vi "Case Structure.vi"() -> ()   [LabVIEW 2020]
panel:
  out "Boolean":bool
  in  "Checkbox":bool
  # "Case Structure"
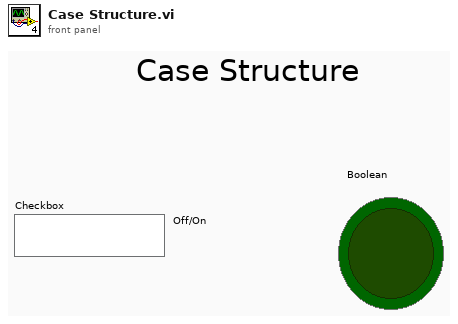
[diagram p1: front panel]
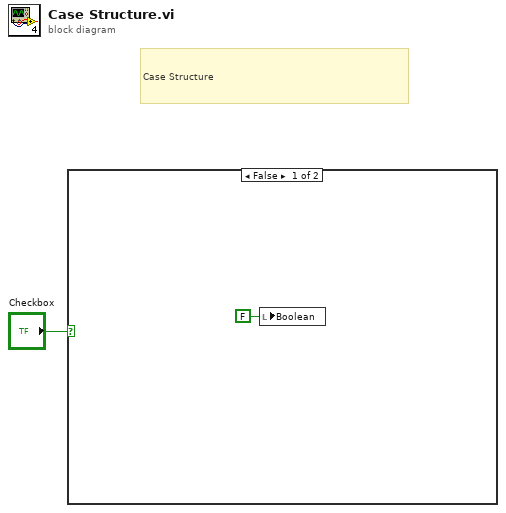
[diagram p0: block diagram]
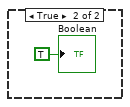
[diagram p2: hidden frame]
diagram:
  # "Case Structure"
  n1 = case shown="False" "Checkbox" {
    frame False {
      n2 = local write "Boolean"(FALSE ("Boolean")) -> ()
    }
    frame True {
      "Boolean" <- TRUE ("Boolean")
    }
  }
